vi "ResMgr-WatchdogThread.vi"(10 "From Who":string, 11 "WatchDogQ":refnum<queue>) -> ()   [LabVIEW 2017, in "Communicable State Machine.lvlib"]
uses:
  Communicable State Machine.lvlib
  ChangeFlag/ChangeFlag-Write.vi
  Utility/Random Change Flag.vi
  ChangeFlag/ChangeFlagDB.vi
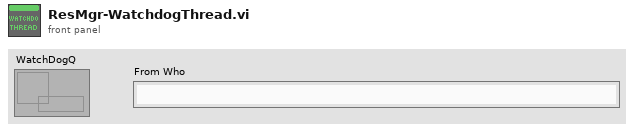
[diagram p1: front panel]
types:
  T1 = cluster{"ResType":string, "RespQ":refnum<queue>, "Parameter":string, "WatchDogQ":refnum<queue>}
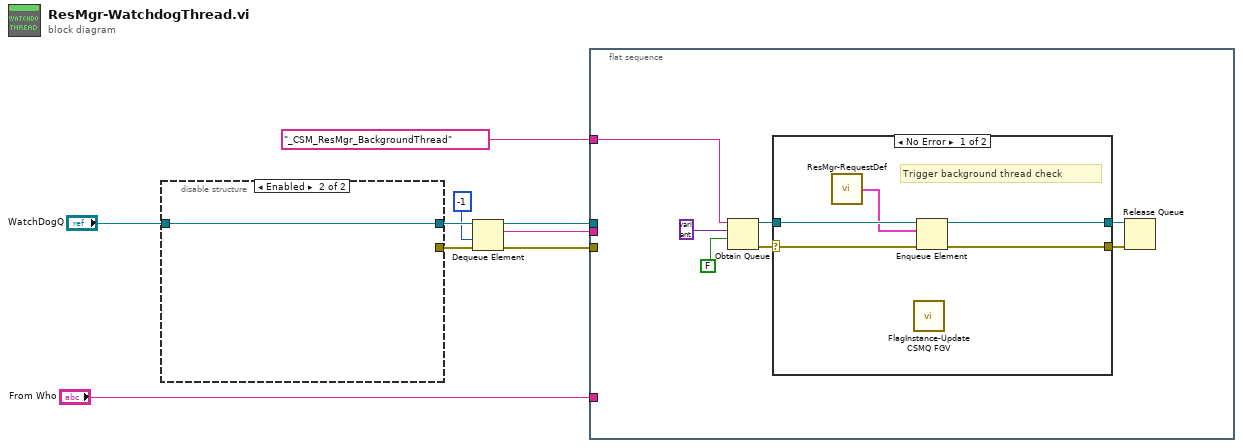
[diagram p0: block diagram]
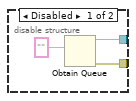
[diagram p3: hidden frame]
diagram:
  n1 = disable-structure shown="Enabled" {
    disable-tunnel: [w11 w13] -> w9
    disable-tunnel: [w10 _] -> w7
    disable-tunnel: "WatchDogQ" -> [_ w13]
    frame Disabled {
      n2 = Obtain Queue(element data type="") -> (queue out=w11:refnum<queue>, error out=w10:errorcluster)  [unwired: 4 in, 1 out]
    }
    frame Enabled {
    }
  }
  n3 = Dequeue Element(queue=w9, timeout in ms (-1)=-1, error in (no error)=w7) -> (queue out=w6:refnum<queue>, element=w2:string, error out=w1:errorcluster)  [unwired: 1 out]
  n4 = flat-sequence {
    tunnel: w6 -> [_]
    tunnel: "_CSM_ResMgr_BackgroundThread" ("name (unnamed)") -> [w15]
    tunnel: "From Who" -> [_]
    tunnel: w2 -> [_]
    tunnel: w1 -> [_]
    frame #0 {
      n5 = Obtain Queue(name (unnamed)=w15, element data type=variant, create if not found? (T)=FALSE) -> (queue out=w18:refnum<queue>, error out=w19:errorcluster)  [unwired: 2 in, 1 out]
      n6 = case shown="No Error" w19 {
        selector: w19 -> [w22 w26]
        tunnel: w18 -> [w25 w27]
        tunnel: [w24 w27] -> w17
        tunnel: [w23 w26] -> w16
        frame No Error {
          # "Trigger background thread check"
          n7 = call "ResMgr-RequestDef.vi"() -> ("ResMgr-RequestDef.ctl"=w21:T1)  [unwired: 2 in]
          n8 = call "FlagInstance-Update CSMQ FGV.vi"() -> ()  [unwired: 10 in, 2 out]
          n9 = Enqueue Element(queue=w25, element=w21, error in (no error)=w22) -> (queue out=w24:refnum<queue>, error out=w23:errorcluster)  [unwired: 1 in, 1 out]
        }
        frame Error {
        }
      }
      n10 = Release Queue(queue=w17, error in (no error)=w16) -> ()  [unwired: 1 in, 3 out]
    }
  }
